vi "histogram.vi"() -> ()   [LabVIEW 2014]
uses:
  <vilib>/Analysis/NI_AALBase.lvlib
panel:
  out "Delta Signal/1st Signal":dbl
  out "variance":dbl=2.5379735179532916e-06 format="%0.6f"
  out "standard deviation":dbl=0.0015931018542306992 format="%0.6f"
  out "Variação %":dbl=0.5566942454415343
  out "max value":dbl=1.3523696381669688
  out "mean":dbl=1.3488164319306033 format="%0.2f"
  out "Signal peak-to-peak":dbl=0.0075285639527740145
  out "Histogram Graph":T1(graph)={"X Values"=[1.3452175024118334, 1.3459703588071108, 1.3467232152023882, 1.3474760715976657, 1.3482289279929431, 1.3489817843882204, 1.3497346407834978, 1.3504874971787753, 1.3512403535740527, 1.3519932099693301], "Histogram: h(x)"=[2, 4, 8, 12, 13, 18, 20, 10, 4, 4]}
  in  "Z-Scan Graph":dbl[](graph)=[1.349038773963978, 1.3484598099859677, 1.3500555695470495, 1.3499940375104709, 1.3497275421169086, 1.345680263895644, 1.34932967543969, 1.3488145738094406, 1.348462082481315, 1.3496520192895591, 1.346893899377366, 1.3520633724602598, 1.346417878426076, 1.3464591153968863, 1.3487775740654004, 1.3523696381669688, 1.3499804620703313, 1.348922829054221, 1.3494990341754884, 1.3503483632152955, 1.3500180472829708, 1.3472611569922834, 1.348381787598058, 1.3479266687083475, 1.3490281786372376, 1.3473406091881939, 1.3458493177302724, 1.3472602689608726, 1.3468598618453005, 1.3489423850122368, 1.346485840615062, 1.3496916460841868, 1.3498930410629413, 1.3518130063926561, 1.3498002430697496, 1.3482814878688023, 1.3512306468469089, 1.3501782324440021, 1.3492445782618014, 1.3509487330354222, 1.3492251950315015, 1.3496093740700836, 1.3505562069101773, 1.3498587084094347, 1.350642151791922, 1.3471617793214554, 1.3495088477039878, 1.3500357308756197, 1.3501763557679956, 1.3509052080741528, 1.3488998356880497, 1.3512134794808177, 1.3476016843837946, 1.3517937758237892, 1.3471616681456446, 1.3475063036985957, 1.34605603439545, 1.348620266438079, 1.34965935264144, 1.3493560455723865, 1.3477188012576051, 1.3490690804966012, 1.3461480431013972, 1.350362090098022, 1.349477912085501, 1.3480412764919396, 1.3492032039296324, 1.3478031260012389, 1.3504674879483154, 1.3498463059947676, 1.3476265172150916, 1.3483926958605044, 1.3484737233321094, 1.3463834562672188, 1.3501375971180647, 1.3507526158919794, 1.34879666489901, 1.3448410742141947, 1.348156532591712, 1.3482027975941948, 1.3474704785864962, 1.3505287284115166, 1.3484296441691266, 1.3452826470962789, 1.3481496299190112, 1.3498904645245258, 1.3481045685202824, 1.3490271110599767, 1.346699260232447, 1.3472503351359735, 1.3492858015119416, 1.3500034530086582, 1.349419770439203, 1.348795761937162, 1.3463921201556102]
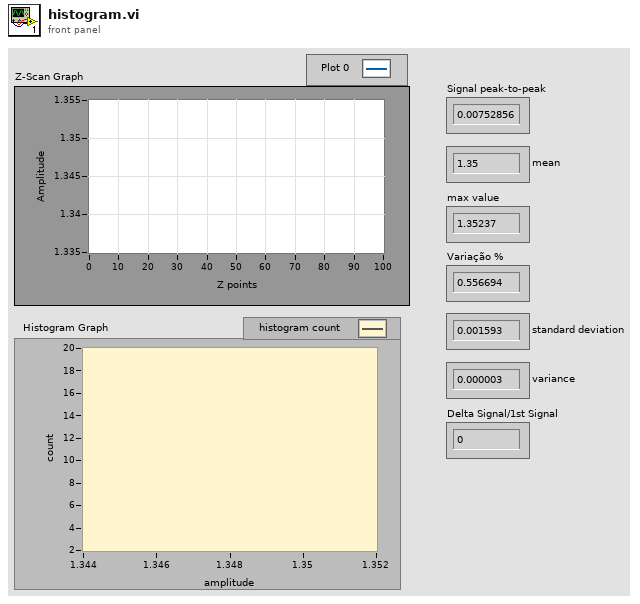
[diagram p1: front panel]
types:
  T1 = cluster{"X Values":dbl[], "Histogram: h(x)":i32[]}
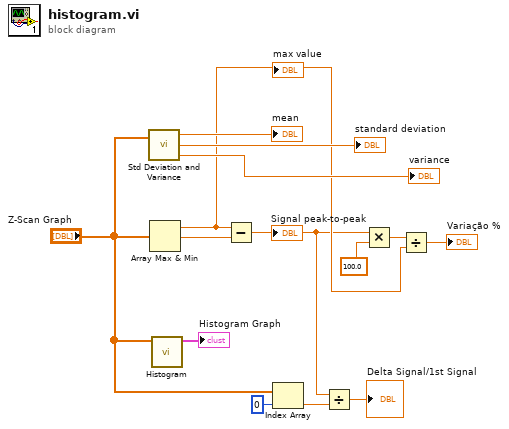
[diagram p0: block diagram]
diagram:
  n1 = call <vilib>:"Std Deviation and Variance.vi"("X"="Z-Scan Graph") -> ("mean"=→"mean":dbl, "standard deviation"=→"standard deviation":dbl, "variance"=→"variance":dbl)  [unwired: 1 in]
  n2 = Array Max & Min(array="Z-Scan Graph") -> (max value=w6:dbl, min value=w13:dbl)  [unwired: 2 out]
  "max value" <- w6
  n3 = call <vilib>:"Histogram.vi"("X"="Z-Scan Graph") -> ("Histogram Graph"=→"Histogram Graph":T1)  [unwired: 7 in, 3 out]
  n4 = Subtract(x=w6, y=w13) -> (x-y=w2:dbl)
  "Signal peak-to-peak" <- w2
  n5 = Index Array(array="Z-Scan Graph", index=0) -> (element=w3:dbl)
  n6 = Divide(x=w2, y=w3) -> (x/y=→"Delta Signal/1st Signal":dbl)
  n7 = Multiply(x=w2, y=100.0) -> (x*y=w11:dbl)
  n8 = Divide(x=w11, y=w6) -> (x/y=→"Variação %":dbl)
